vi "SP Change Trace Orientation on Currently Selected Plot.vi"(2 "Plots Tab Control":refnum<vi>, 3 "Plot Reference":refnum<vi>, 4 "Trace Orientation":enum32{"Overlay", "Split"}(radio)) -> (0 "dup Plot Reference":refnum<vi>)   [LabVIEW 2011]
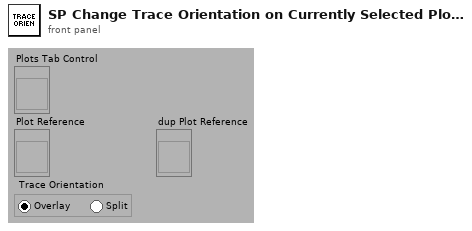
[diagram p1: front panel]
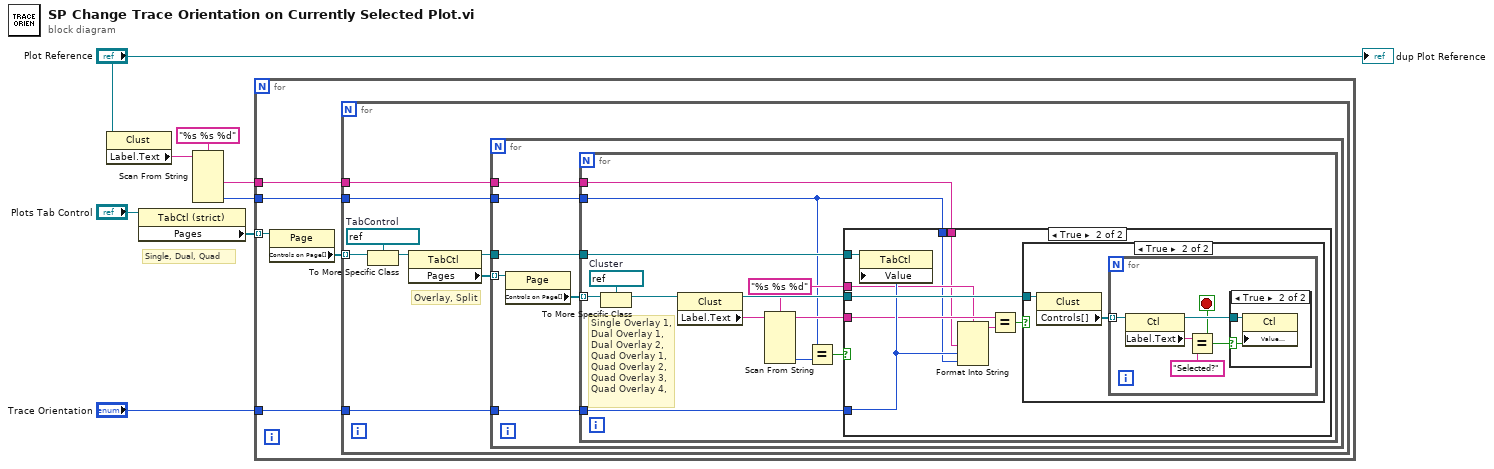
[diagram p0: block diagram]
diagram:
  # "Single, Dual, Quad"
  n1 = property class="Clust"(reference="Plot Reference") -> ("Label.Text"=w2:string)  [unwired: 1 in, 2 out]
  n2 = property class="TabCtl (strict)"(reference="Plots Tab Control") -> ("Pages"=w8:refnum<vi>[])  [unwired: 1 in, 2 out]
  n3 = Scan From String(format string="%s %s %d", input string=w2) -> (output 1=w1:string, output 3=w3:i32)  [unwired: 2 in, 7 out]
  n4 = for {
    tunnel: w8 -> [w13] mode=indexing
    tunnel: "Trace Orientation" -> [w11]
    tunnel: w3 -> [w10]
    tunnel: w1 -> [w9]
    n5 = property class="Page"(reference=w13) -> ("Controls on Page[]"=w12:refnum<vi>[])  [unwired: 1 in, 2 out]
    n6 = for {
      tunnel: w12 -> [w21] mode=indexing
      tunnel: w11 -> [w16]
      tunnel: w10 -> [w15]
      tunnel: w9 -> [w14]
      w20 = refnum<vi> refnum  # TabControl
      # "Overlay, Split"
      n7 = To More Specific Class(target class=w20, reference=w21) -> (specific class reference=w19:refnum<vi>)  [unwired: 1 in, 1 out]
      n8 = property class="TabCtl"(reference=w19) -> (reference out=w17:refnum<vi>, "Pages"=w18:refnum<vi>[])  [unwired: 1 in, 1 out]
      n9 = for {
        tunnel: w18 -> [w27] mode=indexing
        tunnel: w17 -> [w25]
        tunnel: w16 -> [w24]
        tunnel: w15 -> [w23]
        tunnel: w14 -> [w22]
        n10 = property class="Page"(reference=w27) -> ("Controls on Page[]"=w26:refnum<vi>[])  [unwired: 1 in, 2 out]
        n11 = for {
          tunnel: w26 -> [w38] mode=indexing
          tunnel: w25 -> [w37]
          tunnel: w24 -> [w36]
          tunnel: w23 -> [w28]
          tunnel: w22 -> [w29]
          w30 = "%s %s %d" ("format string")
          w39 = refnum<vi> refnum  # Cluster
          # "Single Overlay 1,\nDual Overlay 1,\nDual Overlay 2,\nQuad Overlay 1,\nQuad Overlay 2,\nQuad Overlay 3,\nQuad Overlay 4,"
          n12 = To More Specific Class(target class=w39, reference=w38) -> (specific class reference=w34:refnum<vi>)  [unwired: 1 in, 1 out]
          n13 = property class="Clust"(reference=w34) -> (reference out=w33:refnum<vi>, "Label.Text"=w31:string)  [unwired: 1 in, 1 out]
          n14 = Scan From String(format string=w30, input string=w31) -> (output 3=w32:i32)  [unwired: 2 in, 8 out]
          n15 = Equal?(x=w28, y=w32) -> (x = y?=w35:bool)
          n16 = case shown="True" w35 {
            tunnel: w37 -> [_ w48]
            tunnel: w36 -> [_ w45]
            tunnel: w33 -> [_ w47]
            tunnel: w31 -> [_ w44]
            tunnel: w30 -> [_ w43]
            tunnel: w29 -> [_ w41]
            tunnel: w28 -> [_ w40]
            frame False {
            }
            frame True {
              n17 = property class="TabCtl"(reference=w48, "Value"=w45) -> ()  [unwired: 1 in, 2 out]
              n18 = Format Into String(format string=w43, w41, w45, w40) -> (resulting string=w42:string)  [unwired: 2 in, 1 out]
              n19 = Equal?(x=w44, y=w42) -> (x = y?=w46:bool)
              n20 = case shown="True" w46 {
                tunnel: w47 -> [_ w49]
                frame False {
                }
                frame True {
                  n21 = property class="Clust"(reference=w49) -> ("Controls[]"=w50:refnum<vi>[])  [unwired: 1 in, 2 out]
                  n22 = for {
                    tunnel: w50 -> [w55] mode=indexing
                    stop <- w51 stop-if-true
                    n23 = property class="Ctl"(reference=w55) -> (reference out=w53:refnum<vi>, "Label.Text"=w52:string)  [unwired: 1 in, 1 out]
                    n24 = Equal?(x=w52, y="Selected?") -> (x = y?=w51:bool)
                    n25 = case shown="True" w51 {
                      selector: w51 -> [_ w56]
                      tunnel: w53 -> [_ w57]
                      frame False {
                      }
                      frame True {
                        n26 = property class="Ctl"(reference=w57, "Value (Signaling)"=w56) -> ()  [unwired: 1 in, 2 out]
                      }
                    }
                  }
                }
              }
            }
          }
        }
      }
    }
  }
  "dup Plot Reference" <- "Plot Reference"
